vi "subSetDigStates_NW348.vi"(6 "wait (sec)":dbl, 8 "Error in (no error)":errorcluster, 10 "Digital line array":tag[](array[tag]), 11 "Digital state array":bool[](array[boolean])) -> (0 "Error out":errorcluster)   [LabVIEW 2012]
uses:
  <vilib>/DAQmx/write.llb/DAQmx Write (Digital 1D Bool NChan 1Samp 1Line).vi
  <vilib>/DAQmx/create/channels.llb/DAQmx Create Channel (DO-Digital Output).vi
  <vilib>/DAQmx/miscellaneous.llb/DAQmx Fill In Error Info.vi
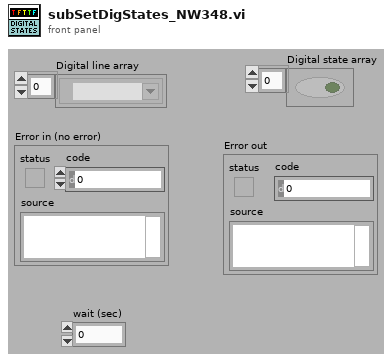
[diagram p1: front panel]
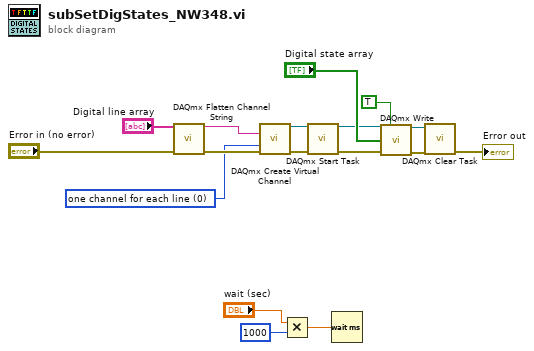
[diagram p0: block diagram]
diagram:
  w11 = 0 items=["one channel for each line", "one channel for all lines"] ("line grouping")
  n1 = call <vilib>:"DAQmx Flatten Channel String.vi"("names in"="Digital line array", "error in"="Error in (no error)") -> ("names out"=w10:string, "error out"=w17:errorcluster)  [unwired: 12 out]
  n2 = call-poly <vilib>:"DAQmx Create Virtual Channel.vi"("lines"=w10, "line grouping"=w11, "error in"=w17) -> ("task out"=w13:refnum<k21>, "error out"=w12:errorcluster)  [unwired: 2 in, 9 out]
  n3 = Multiply(x="wait (sec)", y=u32 1000) -> (x*y=w1:dbl)
  n4 = call <vilib>:"DAQmx Start Task.vi"("task/channels in"=w13, "error in"=w12) -> ("task out"=w9:refnum<k21>, "error out"=w8:errorcluster)  [unwired: 12 out]
  n5 = Wait (ms)(milliseconds to wait=w1) -> ()  [unwired: 1 out]
  n6 = call-poly <vilib>:"DAQmx Write.vi"("task/channels in"=w9, "auto start"=TRUE, "data"="Digital state array", "error in"=w8) -> ("task out"=w6:refnum<k21>, "error out"=w5:errorcluster)  [unwired: 10 out]
  n7 = call <vilib>:"DAQmx Clear Task.vi"("task in"=w6, "error in"=w5) -> ("error out"=→"Error out":errorcluster)  [unwired: 13 out]
